vi "RPM Band--constant.vi"() -> (0 "RPM Band":i16=10)   [LabVIEW 2024, in "Auto Modo.lvlib"]
uses:
  Auto Modo.lvlib
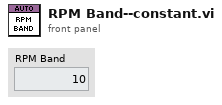
[diagram p1: front panel]
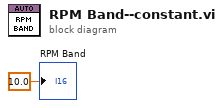
[diagram p0: block diagram]
diagram:
  "RPM Band" <- 10.0
